vi "parseSerialData.vi"(8 "error in (no error)":errorcluster, 10 "serialData":string="M0,-000.0154,+000.0685", 11 "DistanceGauge in":refnum<class "DistanceGauge.lvclass">) -> (0 "error out":errorcluster, 2 "dataArray":dbl[unit][](array[numeric]), 3 "DistanceGauge out":refnum<class "DistanceGauge.lvclass">)   [LabVIEW 2013, in "DistanceGauge.lvclass"]
uses:
  DistanceGauge.lvclass
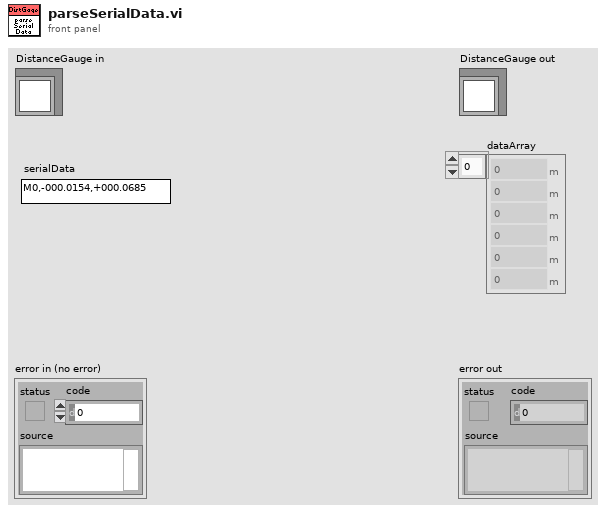
[diagram p1: front panel]
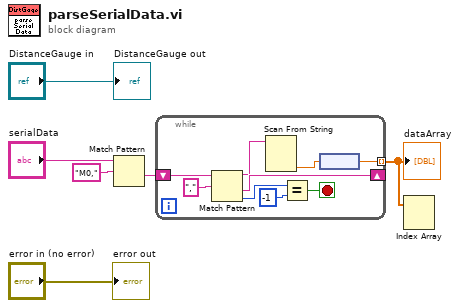
[diagram p0: block diagram]
diagram:
  n1 = Match Pattern(string="serialData", regular expression="M0,") -> (after substring=w2:string)  [unwired: 1 in, 3 out]
  n2 = while {
    shift-right: [w13] -> _
    shift-left: w2 -> [w15]
    tunnel: [w7] -> w1 mode=indexing
    stop <- w10 stop-if-true
    n3 = Match Pattern(string=w15, regular expression=",") -> (before substring=w9:string, after substring=w13:string, offset past match=w12:i32)  [unwired: 1 in, 1 out]
    n4 = Scan From String(input string=w9) -> (output 1=w8:dbl)  [unwired: 4 in, 3 out]
    n5 = Equal?(x=w12, y=-1) -> (x = y?=w10:bool)
    n6 = node(w8) -> (w7:dbl[unit])
  }
  "dataArray" <- w1
  n7 = Index Array(array=w1) -> ()  [unwired: 2 in, 2 out]
  "error out" <- "error in (no error)"
  "DistanceGauge out" <- "DistanceGauge in"
